vi "Helper - Export - Triangle.vi"() -> (3 "Triangle with Noise":dbl[](array[numeric]))   [LabVIEW 2023]
doc: "Generates a Triangle signal with noise."
panel:
  # "Generates a Triangle signal with noise."
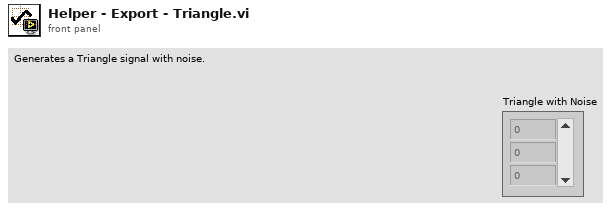
[diagram p1: front panel]
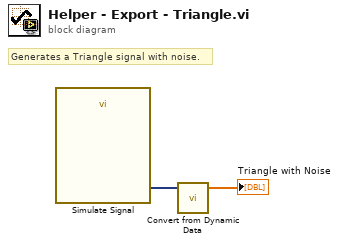
[diagram p0: block diagram]
diagram:
  # "Generates a Triangle signal with noise."
  n1 = call "Simulate Signal"() -> ("Triangle with Uniform Noise"=w2:dynamicdata)  [unwired: 14 in, 1 out]
  n2 = call "Convert from Dynamic Data"("Dynamic Data Type"=w2) -> ("Array"=→"Triangle with Noise":dbl[])  [unwired: 3 in]
